vi "Test Broadcast Unfiltered Debug Log Not Filtered by Process.vi"(8 "error in (no error)":errorcluster, 11 "Test Case In":refnum<class "Debugger Test.lvclass">) -> (0 "error out":errorcluster, 3 "Test Case Out":refnum<class "Debugger Test.lvclass">)   [LabVIEW 2020, in "Debugger Test.lvclass"]
uses:
  Debugger Test.lvclass
  C:/Program Files (x86)/National Instruments/LabVIEW 2020/vi.lib/Astemes/LUnit/Test Case.lvclass
  source/Debugger/Debugger.lvclass
  C:/Users/anton/Documents/GitHub/triarc-debugger/source/Process/Debug Process.lvclass
  source/Debug Data/Raw Debug Data.ctl
  source/Process/Debug Process.lvclass/Debug Process.ctl
  <vilib>/Astemes/LUnit/Test Case.lvclass/Test Case.ctl
  <vilib>/Astemes/LUnit/LUnit Assertion Result.lvclass/LUnit Assertion Result.ctl
  <vilib>/Astemes/LUnit/LUnit Test Case Result.lvclass/LUnit Test Case Result.ctl
  <vilib>/Astemes/LUnit/LUnit Method Result.lvclass/LUnit Method Result.ctl
  01074fa8-ee8a-411d-bc8b-fc92c4f90959.vi
  source/Process/Public/Lifecycle/Get Lifecycle State.vi
  source/Process/Private/SubVIs/Wait for finish.vi
  source/Process/Protected/Messaging/Enqueue Message.vi
  source/Process/Private/SubVIs/Set Lifecycle State.vi
  <vilib>/Astemes/LUnit/Palette/Pass.vi
  <vilib>/Astemes/LUnit/Palette/Fail.vi
  <vilib>/Astemes/LUnit/Compare Variants.vi
  <vilib>/Astemes/LUnit/Describe Comparison.vi
  <vilib>/Astemes/LUnit/Set Assertion Type.vi
  <vilib>/Utility/error.llb/Clear Errors.vi
  <vilib>/Astemes/LUnit/Add test result.vi
  <vilib>/Astemes/LUnit/LUnit Write Passed.vi
  <vilib>/Astemes/LUnit/LUnit Write Message.vi
  <vilib>/Astemes/LUnit/LUnit Write Description.vi
  <vilib>/Astemes/LUnit/Variant to string.vi
  <vilib>/Astemes/LUnit/LUnit Write Assertion Type.vi
  <vilib>/Astemes/LUnit/LUnit Record Assertion Result.vi
  <vilib>/Astemes/LUnit/LUnit Aggregate Assertion Results.vi
  <vilib>/Astemes/LUnit/Assertion Result/LUnit Read Status.vi
  <vilib>/Astemes/LUnit/LUnit Read Message.vi
  <vilib>/Astemes/LUnit/LUnit Read Description.vi
  <vilib>/Astemes/LUnit/Method Result/LUnit Merge Status.vi
  <vilib>/Astemes/LUnit/LUnit Concatenate result strings.vi
  <vilib>/Utility/error.llb/Error Cluster From Error Code.vi
  <vilib>/Utility/Data Type/Get Type Information.vi
  <vilib>/Utility/LVClass/Get LV Class Name.vi
  <vilib>/Astemes/LUnit/LUnit Assertion Result.lvclass
  source/Process/Debug Process.lvclass
  Debugger Test.lvclass/Debugger Test.ctl
  source/Debug Data/Debug Data.lvclass
  C:/Users/anton/Documents/GitHub/triarc-debugger/source/Debugger/Debugger.lvclass
  C:/Users/anton/Documents/GitHub/triarc-debugger/source/Debug Data Event/Debug Data Listener.lvclass
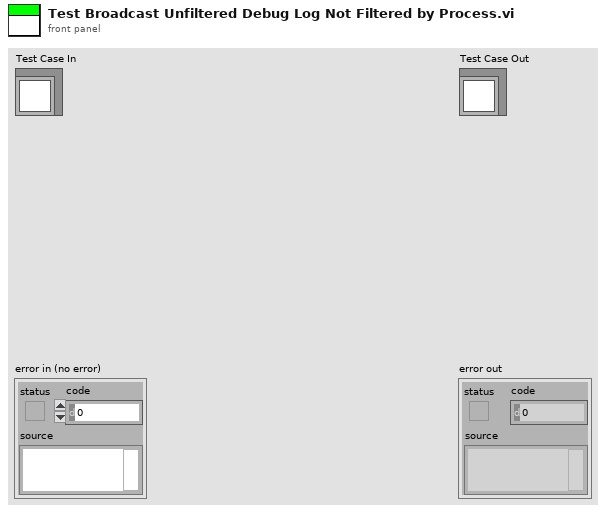
[diagram p1: front panel]
types:
  T1 = typedef "Debug Data.lvclass/Raw Debug Data.ctl" = cluster{"Action":string, "Call Chain":string, "Process":string, "Message":string, "Message Data":variant, "Time":u32}
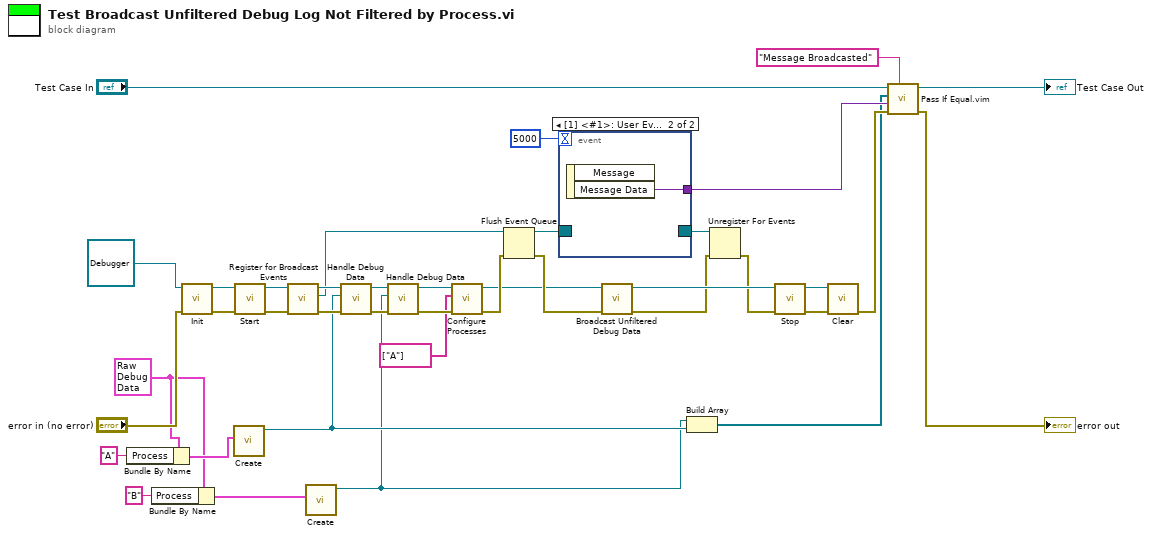
[diagram p0: block diagram]
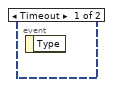
[diagram p2: hidden frame]
diagram:
  w8 = T1 {"Action"="", "Call Chain"="", "Process"="", "Message"="", "Message Data"=variant, "Time"=0} ("Debug Data Cluster")
  n1 = Bundle By Name(cluster=w8, "Process"="A") -> (w15:T1)
  n2 = Bundle By Name(cluster=w8, "Process"="B") -> (w9:T1)
  n3 = call-dynamic "Init.vi"("error in (no error)"="error in (no error)", "Process In"=refnum<class "Debugger.lvclass"> refnum ("Debug Data Event In 2")) -> ("error out"=w35:errorcluster, "Process Out"=w36:refnum<class "Debugger.lvclass">)  [unwired: 8 in]
  n4 = call "Create.vi"("Debug Data Cluster"=w15) -> ("Debug Data out"=w21:refnum<class "Debug Data.lvclass">)  [unwired: 9 in, 1 out]
  n5 = call "Start.vi"("error in (no error)"=w35, "Process In"=w36) -> ("error out"=w33:errorcluster, "Process Out"=w34:refnum<class "Debugger.lvclass">)  [unwired: 7 in, 1 out]
  n6 = call "Register for Broadcast Events.vi"("error in (no error)"=w33, "Process In"=w34) -> ("error out"=w32:errorcluster, "Event Registration Refnum Out"=w17:refnum<event-registration>, "Process Out"=w28:refnum<class "Debugger.lvclass">)  [unwired: 7 in]
  n7 = call "Create.vi"("Debug Data Cluster"=w9) -> ("Debug Data out"=w3:refnum<class "Debug Data.lvclass">)  [unwired: 9 in, 1 out]
  n8 = call-dynamic "Handle Debug Data.vi"("error in (no error)"=w32, "Debug Data.lvclass"=w21, "Debug Data Event In"=w28) -> ("error out"=w12:errorcluster, "Debug Data Event Out"=w13:refnum<class "Debugger.lvclass">)  [unwired: 7 in]
  n9 = call-dynamic "Handle Debug Data.vi"("error in (no error)"=w12, "Debug Data.lvclass"=w3, "Debug Data Event In"=w13) -> ("error out"=w11:errorcluster, "Debug Data Event Out"=w6:refnum<class "Debugger.lvclass">)  [unwired: 7 in]
  n10 = call "Configure Processes.vi"("error in (no error)"=w11, "Processes"=string[] ["A"], "Debugger In"=w6) -> ("error out"=w7:errorcluster, "Debugger Out"=w5:refnum<class "Debugger.lvclass">)  [unwired: 7 in]
  n11 = Flush Event Queue(0:w17, 3:w7) -> (8:w16:refnum<event-registration>, 11:w18:errorcluster)  [unwired: 4 in, 1 out]
  n12 = event shown="[1] <#1>: User Event" {
    selector: w16 -> [_ _]
    dyn-events: [_ _] -> w23
    timeout: 5000 -> [_ _]
    tunnel: [_ w40] -> w20
    event Timeout {
      n13 = event-data() -> ()  [unwired: 1 in, 1 out]
    }
    event User Event {
      n14 = event-data() -> ("Message Data"=w40:variant)  [unwired: 1 in, 1 out]
    }
  }
  n15 = call "Broadcast Unfiltered Debug Data.vi"("error in (no error)"=w18, "Debugger in"=w5) -> ("error out"=w2:errorcluster, "Debugger out"=w31:refnum<class "Debugger.lvclass">)  [unwired: 8 in]
  n16 = Build Array(w3, w21) -> (w19:refnum<class "Debug Data.lvclass">[])
  n17 = Unregister For Events(event registration refnum=w23, error in=w2) -> (error out=w1:errorcluster)
  n18 = call "Stop.vi"("error in (no error)"=w1, "Process In"=w31) -> ("error out"=w29:errorcluster, "Process Out"=w30:refnum<class "Debugger.lvclass">)  [unwired: 7 in, 1 out]
  n19 = call-dynamic "Clear.vi"("error in (no error)"=w29, "Process In"=w30) -> ("error out"=w25:errorcluster)  [unwired: 9 in]
  n20 = call "Pass If Equal.vim"("Description"="Message Broadcasted", "error in (no error)"=w25, "Actual"=w20, "Expected"=w19, "LUnit Test Case In"="Test Case In") -> ("error out"=→"error out":errorcluster, "LUnit Test Case Out"=→"Test Case Out":refnum<class "Debugger Test.lvclass">)  [unwired: 5 in]
